vi "ReadSensorValues_v1.2.vi"(2 "VISA resource name":refnum<visa-resource-name>, 3 "Sensor type":T1) -> ()   [LabVIEW 2012]
uses:
  <vilib>/nican/nicantsk.llb/CAN Interface.ctl
  SensorTypes.ctl
  SensorStates.ctl
  <vilib>/nican/nicantsk.llb/CAN Task Reference.ctl
  <vilib>/nican/nicantsk.llb/CAN Mode.ctl
  globalVariables.vi
  <vilib>/Utility/file.llb/Write To Spreadsheet File (string).vi
  <vilib>/nican/nicantsk.llb/CAN Read Multi Chan Single Samp 1D Dbl.vi
  <instrlib>/Agilent 34970/Agilent 34970.lvlib
panel:
  in  "Cancel Measurement":bool
  out "new data":bool
  out "running":bool
  out "Sample number":i32
  in  "CAN Interface":T2 items=["CAN0"=0, "CAN1"=1, "CAN2"=2, "CAN3"=3, "CAN4"=4, "CAN5"=5, "CAN6"=6, "CAN7"=7, "CAN8"=8, "CAN9"=9, "CAN10"=10, "CAN11"=11, "CAN12"=12, "CAN13"=13, "CAN14"=14, "CAN15"=15, "CAN16"=16, "CAN17"=17, "CAN18"=18, "CAN19"=19, "CAN20"=20, "CAN21"=21, "CAN22"=22, "CAN23"=23, "CAN24"=24, "CAN25"=25, "CAN26"=26, "CAN27"=27, "CAN28"=28, "CAN29"=29, "CAN30"=30, "CAN31"=31, "CAN32"=32, "CAN33"=33, "CAN34"=34, "CAN35"=35, "CAN36"=36, "CAN37"=37, "CAN38"=38, "CAN39"=39, "CAN40"=40, "CAN41"=41, "CAN42"=42, "CAN43"=43, "CAN44"=44, "CAN45"=45, "CAN46"=46, "CAN47"=47, "CAN48"=48, "CAN49"=49, "CAN50"=50, "CAN51"=51, "CAN52"=52, "CAN53"=53, "CAN54"=54, "CAN55"=55, "CAN56"=56, "CAN57"=57, "CAN58"=58, "CAN59"=59, "CAN60"=60, "CAN61"=61, "CAN62"=62, "CAN63"=63, "MAX default"=64, "CAN256 (Virtual)"=256, "CAN257 (Virtual)"=257]
  out "Error Flag":bool
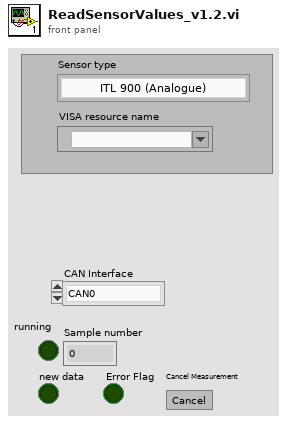
[diagram p1: front panel]
types:
  T1 = typedef "SensorTypes.ctl" = enum16{"ITL 900 (Analogue)", "CAB 300-C SP3 (CAN)", "xyz TODO (PWM)", "xyz TODO (LIN)", "xyz TODO (Analogue)"}
  T2 = typedef "CAN Interface.ctl" = u16
  T3 = typedef "SensorStates.ctl" = enum16{"init", "measure", "terminate"}
  T4 = cluster{"Include Alarm Data F:(No)":bool, "Include Channel # (F:No)":bool, "Include Time (F:No)":bool, "Include Units (F:No)":bool}
  T5 = cluster{"Aperture Value (.4)":dbl, "Aperture (1:Minimum)":u16, "NPLC (1)":u16, "Bandwidth (3 Hz)":u16, "Input Impedance (F:Fixed)":bool, "Integration Time (F:Aperture)":bool}
  T6 = enum16{"100 mV", "1 V", "10 V", "100 V", "300 V", "Minimum", "Maximum"}
  T7 = enum16{"Bus", "Immediate", "External", "Alarm 1", "Alarm 2", "Alarm 3", "Alarm 4", "Timer"}
  T8 = cluster{"Timeout Value (10000)":u32, "Baud Rate (57600)":enum16{"1200", "2400", "4800", "9600", "19200", "38400", "57600", "115200"}, "Flow Control (1:XON/XOFF)":enum16{"None", "XON / XOFF", "RTS / CTS", "DTR / DSR"}}
  T9 = typedef "CAN Task Reference.ctl" = u32
  T10 = enum16{"Remote Trigger", "Immediate Trigger", "Wait for Trigger", "Abort Scan"}
  T11 = typedef "CAN Mode.ctl" = u16
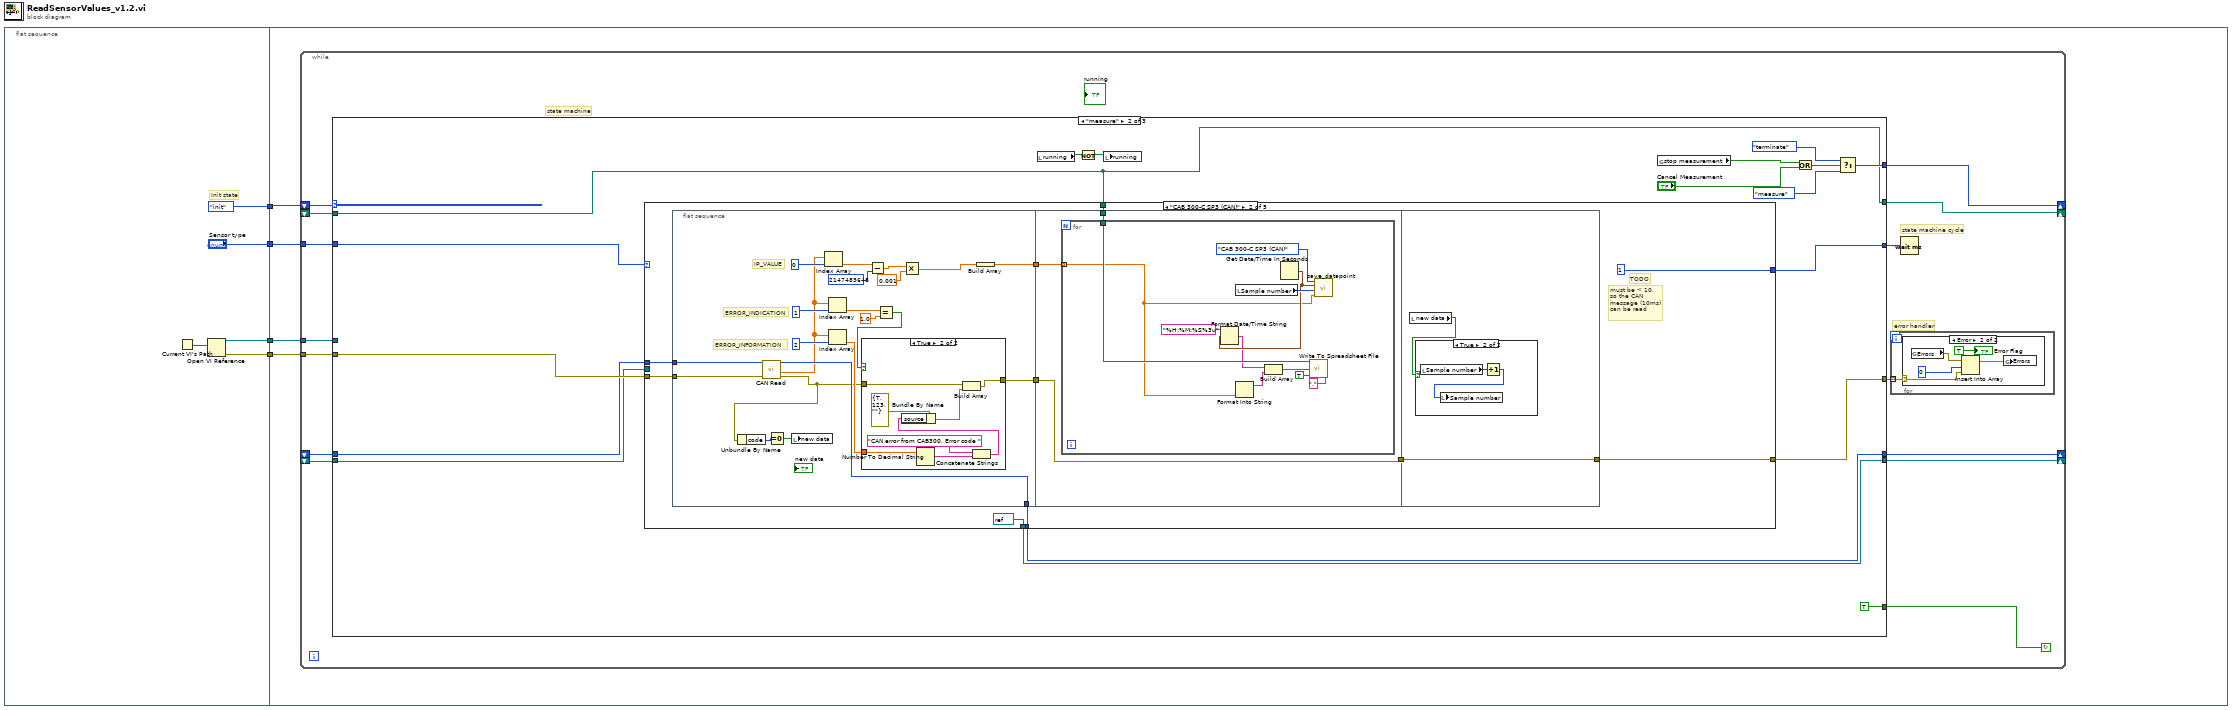
[diagram p0: block diagram]
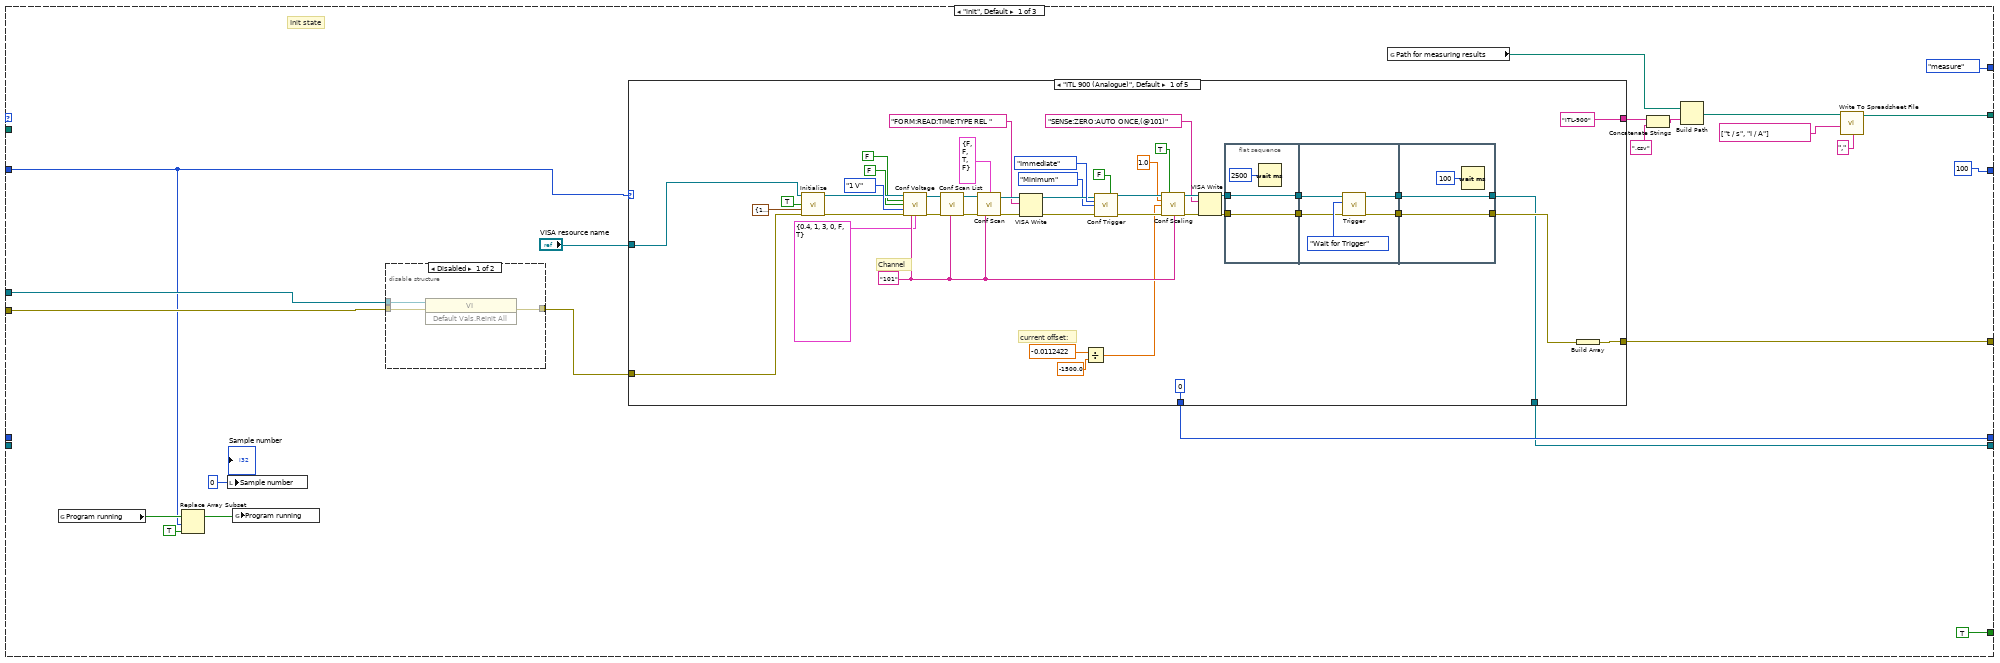
[diagram p3: hidden frame]
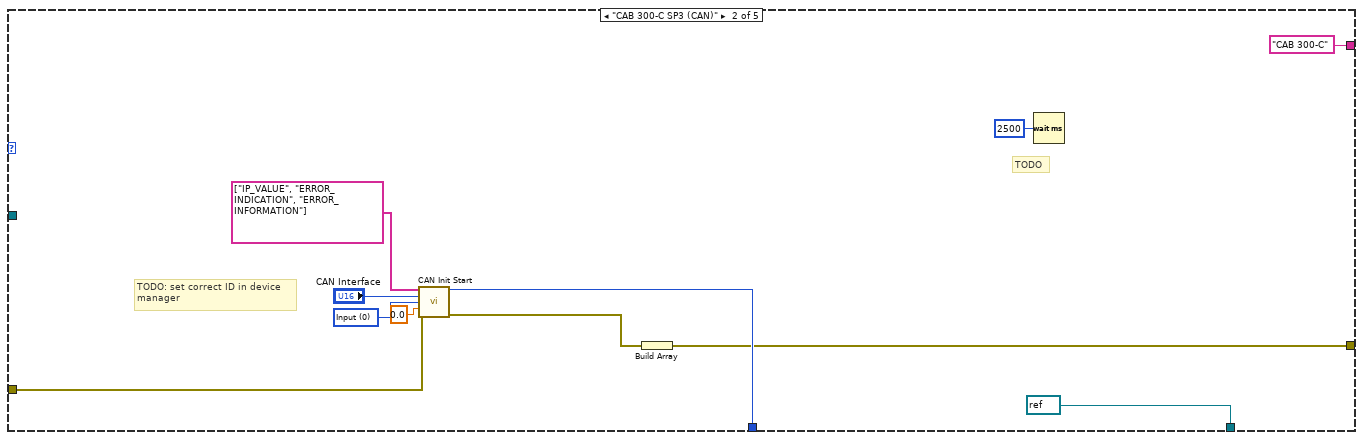
[diagram p5: hidden frame]
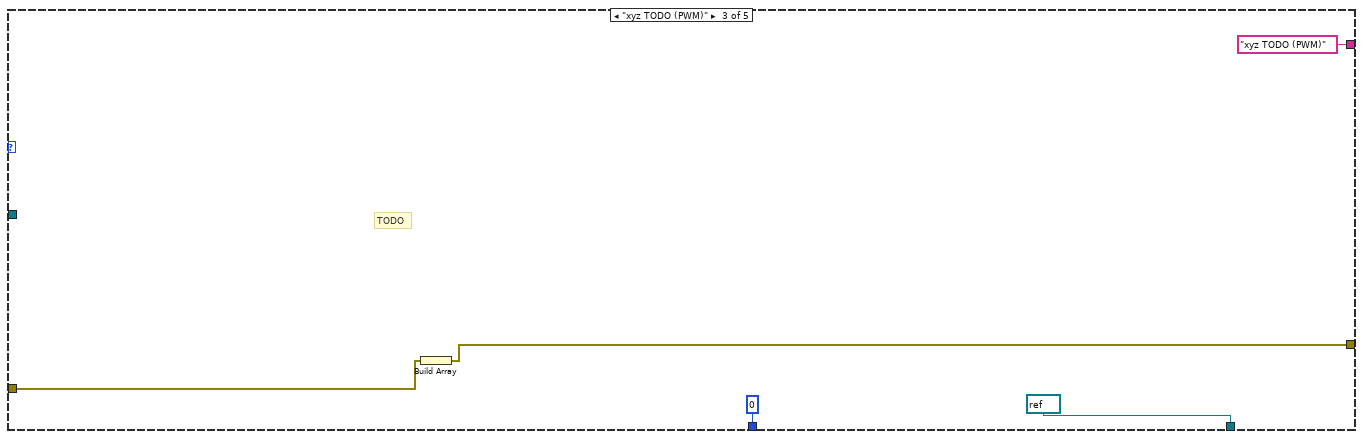
[diagram p6: hidden frame]
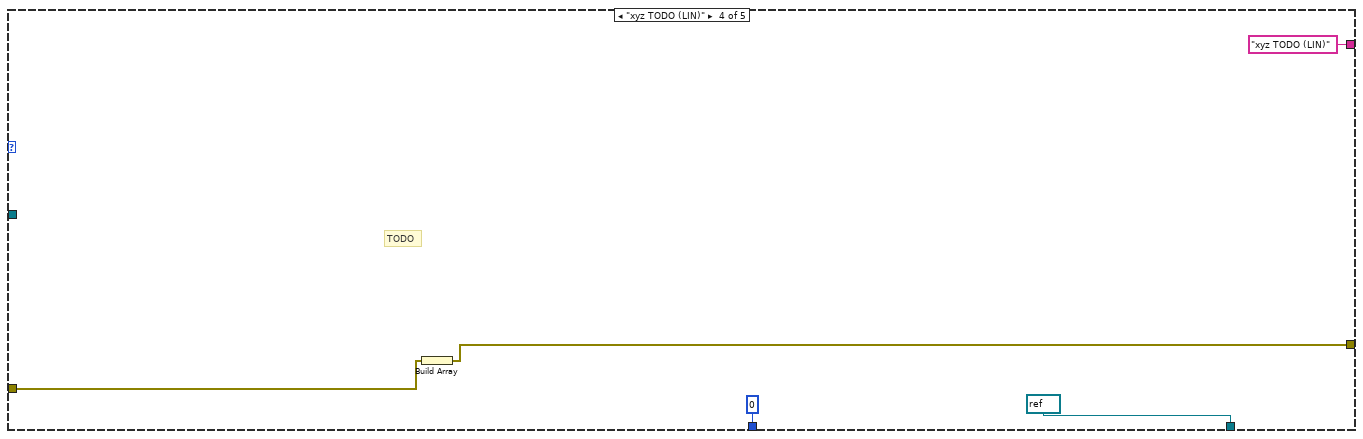
[diagram p7: hidden frame]
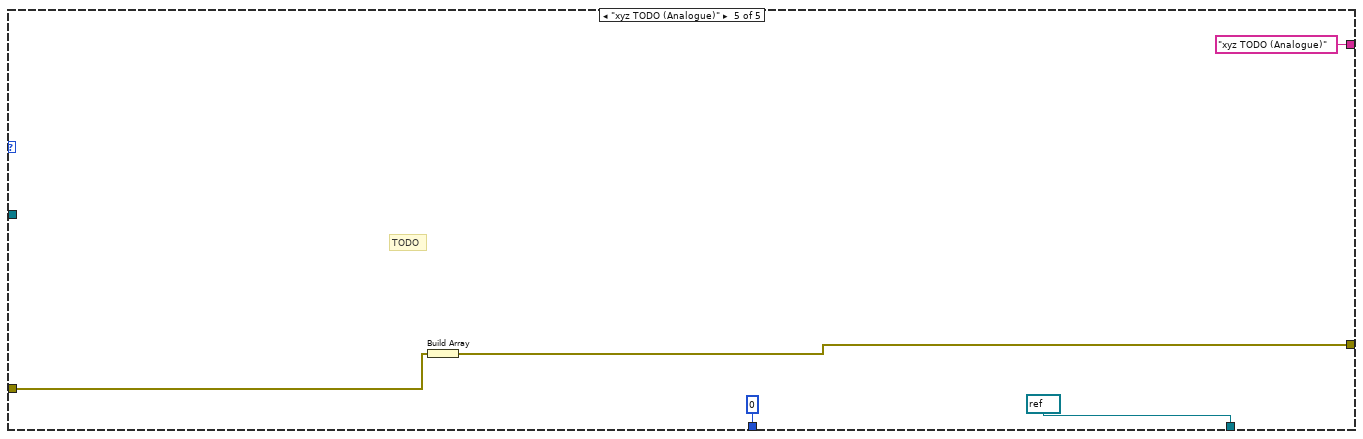
[diagram p8: hidden frame]
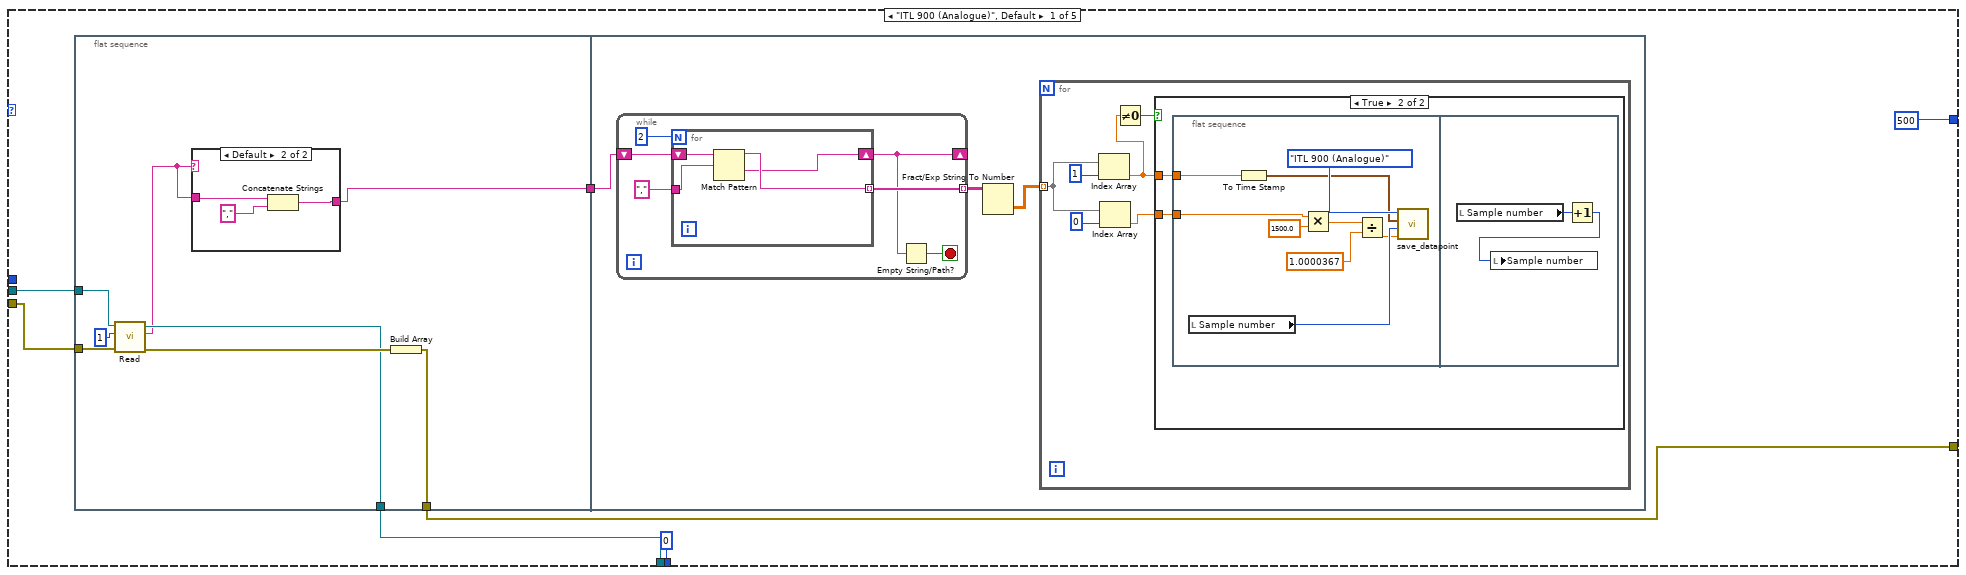
[diagram p9: hidden frame]
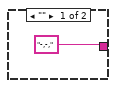
[diagram p10: hidden frame]
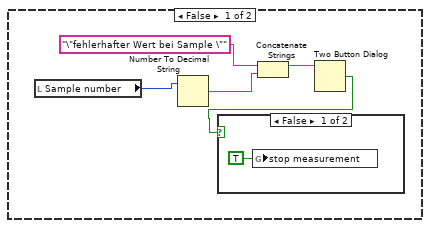
[diagram p11: hidden frame]
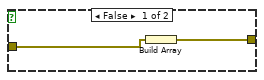
[diagram p13: hidden frame]
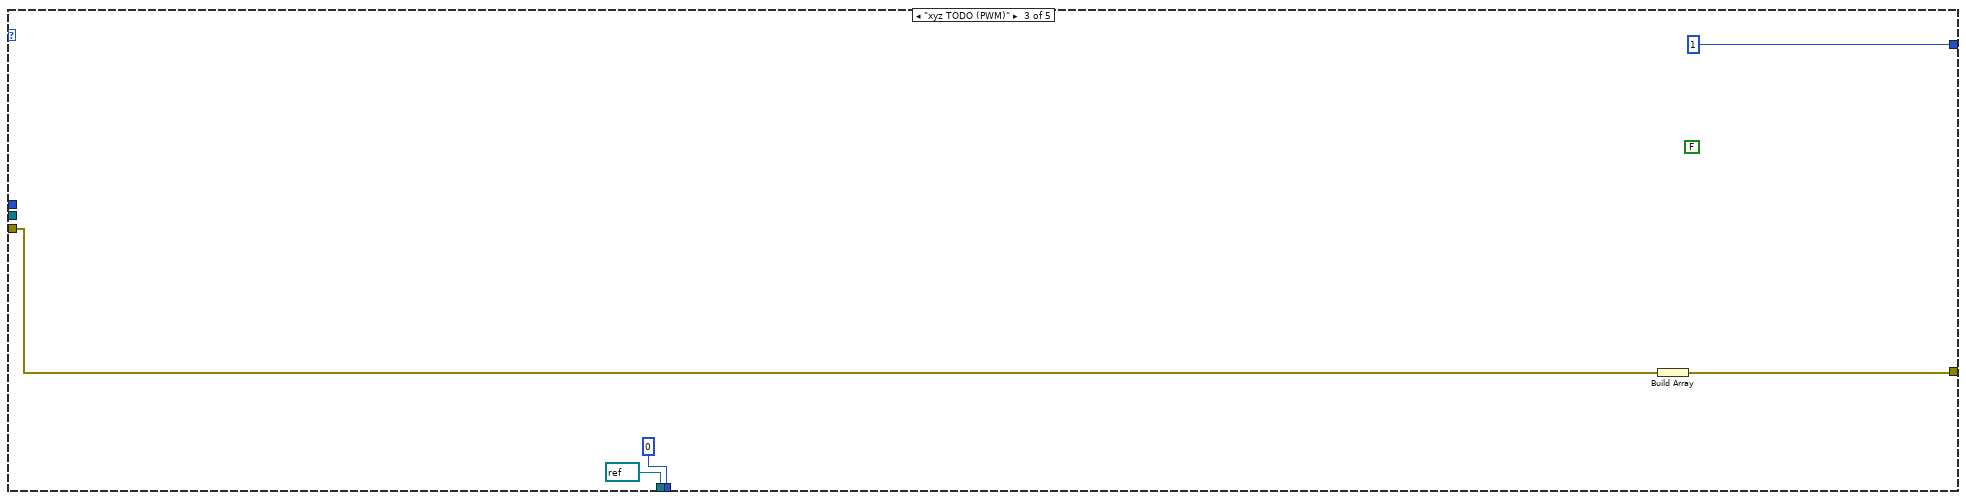
[diagram p15: hidden frame]
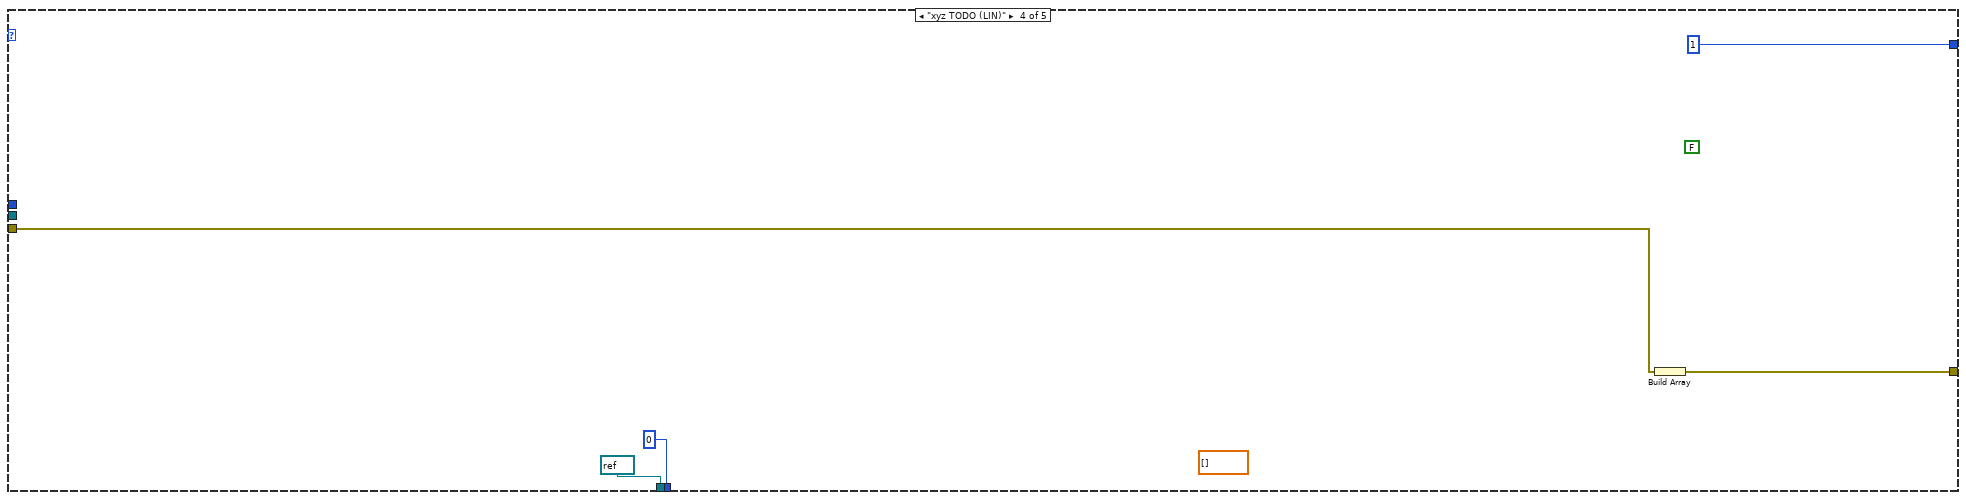
[diagram p16: hidden frame]
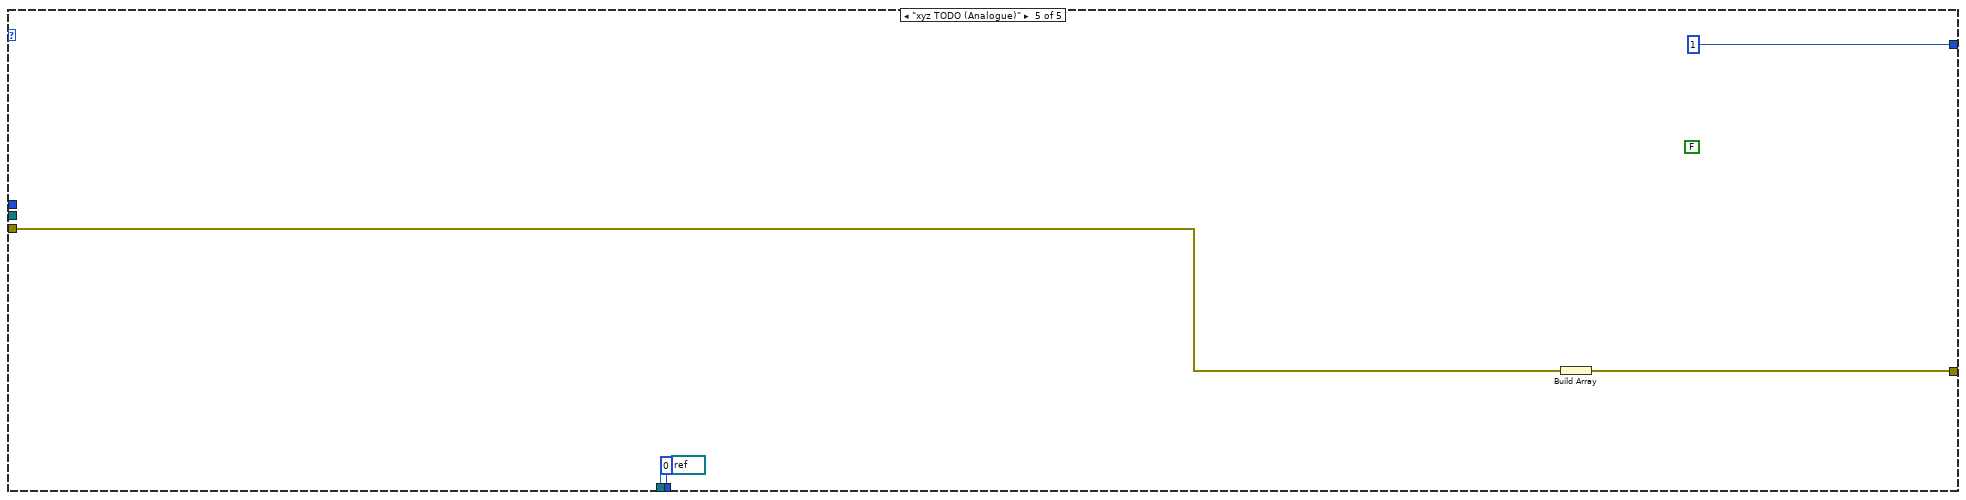
[diagram p17: hidden frame]
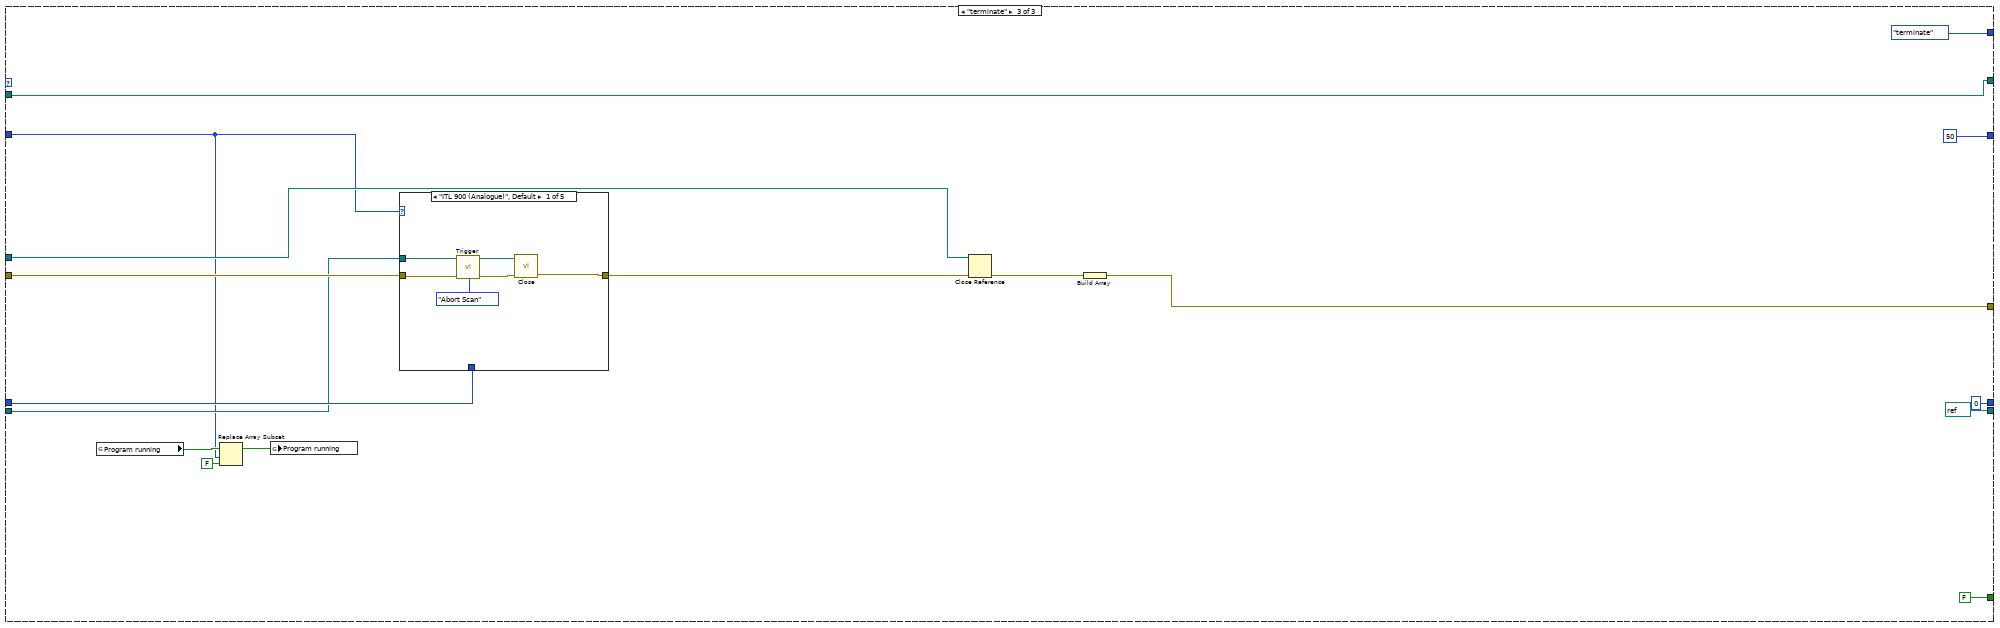
[diagram p18: hidden frame]
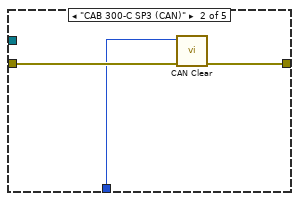
[diagram p19: hidden frame]
diagram:
  n1 = flat-sequence {
    tunnel: [SensorStates."init" ("States IEEE-488")] -> w4
    tunnel: [w9] -> w3
    tunnel: [w8] -> w2
    tunnel: ["Sensor type"] -> w1
    tunnel: w4 -> [w11]
    tunnel: w3 -> [w13]
    tunnel: w2 -> [w12]
    tunnel: w1 -> [w10]
    frame #0 {
      # "Init state"
      n2 = Current VI's Path() -> (path=w7:path)
      n3 = Open VI Reference(vi path=w7) -> (vi reference=w9:refnum<vi>, error out=w8:errorcluster)  [unwired: 2 in, 3 out]
    }
    frame #1 {
      n4 = while {
        tunnel: w13 -> [w26]
        tunnel: w12 -> [w25]
        shift-right: [w23] -> _
        shift-left: w11 -> [w24]
        shift-right: [w22] -> _
        shift-left: _ -> [w21]
        tunnel: w10 -> [w19]
        shift-right: [w18] -> _
        shift-left: _ -> [w17]
        shift-right: [w15] -> _
        shift-left: _ -> [w14]
        stop <- w16 continue-if-true
        # "state machine"
        # "error handler"
        # "state machine cycle"
        n5 = case shown="\"measure\"" w24 {
          tunnel: [u32 100 ("milliseconds to wait") w143 u32 50 ("milliseconds to wait")] -> w27
          tunnel: w26 -> [w54 _ w300]
          tunnel: w25 -> [w55 w156 w304]
          tunnel: [SensorStates."measure" ("States IEEE-488") w157 SensorStates."terminate" ("States IEEE-488")] -> w23
          tunnel: [w52 w150 T9 0 ("task reference out")] -> w22
          tunnel: w21 -> [_ w151 w303]
          tunnel: [w50 w152 w302] -> w20
          tunnel: w19 -> [w42 w144 w292]
          tunnel: [TRUE TRUE FALSE] -> w16
          tunnel: [w46 w145 refnum<visa-resource-name> refnum ("VISA Resource Name Out")] -> w18
          tunnel: w17 -> [_ w146 w297]
          tunnel: [w37 w142 w291] -> w15
          tunnel: w14 -> [_ w142 w291]
          frame "init", Default {
            # "Init state"
            n6 = global read "globalVariables.vi" "Program running"() -> (w45:bool[])
            n7 = Replace Array Subset(array=w45, new element=TRUE ("new element/subarray"), index=w42) -> (w44:bool[])
            n8 = local write "Sample number"(0 ("Sample number")) -> ()
            n9 = global write "globalVariables.vi" "Program running"(w44) -> ()
            n10 = disable-structure shown="Disabled" {
              disable-tunnel: w55 -> [w59 _]
              disable-tunnel: w54 -> [w58 _]
              disable-tunnel: [w57 _] -> w51
              frame Disabled {
                n11 = invoke class="VI" method="Default Vals.Reinit All"(reference=w58, error in=w59) -> (error out=w57:errorcluster)  [unwired: 1 in, 2 out]
              }
              frame Enabled {
              }
            }
            n12 = case shown="\"ITL 900 (Analogue)\", Default" w42 {
              tunnel: [T9 0 ("task reference out") w122 T9 0 ("task reference out") T9 0 ("task reference out") T9 0 ("task reference out")] -> w52
              tunnel: w51 -> [w71 w121 w130 w135 w141]
              tunnel: [w104 w119 w131 w136 w140] -> w50
              tunnel: "VISA resource name" -> [w64 _ _ _ _]
              tunnel: [w69 refnum<visa-resource-name> refnum ("VISA Resource Name Out") refnum<visa-resource-name> refnum ("VISA Resource Name Out") refnum<visa-resource-name> refnum ("VISA Resource Name Out") refnum<visa-resource-name> refnum ("VISA Resource Name Out")] -> w46
              tunnel: ["ITL-900" ("name or relative path") "CAB 300-C" ("name or relative path") "xyz TODO (PWM)" ("name or relative path") "xyz TODO (LIN)" ("name or relative path") "xyz TODO (Analogue)" ("name or relative path")] -> w36
              frame "ITL 900 (Analogue)", Default {
                w77 = "101" ("Channel List (Volt.)")
                # "current offset:"
                # "Channel"
                n13 = call <instrlib>:"Initialize.vi"("VISA Resource Name"=w64, "Reset (T: Reset)"=TRUE, "Serial Port Configuration"=T8 {"Timeout Value (10000)"=10000, "Baud Rate (57600)"=enum."57600", "Flow Control (1:XON/XOFF)"=enum."XON / XOFF"}, "error in (no error)"=w71) -> ("VISA Resource Name Out"=w98:refnum<visa-resource-name>, "error out"=w95:errorcluster)  [unwired: 10 in]
                n14 = call <instrlib>:"Conf Voltage.vi"("VISA Resource Name"=w98, "AC/DC (F:DC)"=FALSE, "Autorange? (F:Off)"=FALSE, "Range (6:Max)"=T6."1 V" ("Range (Volt.)"), "error in (no error)"=w95, "Channel List (empty)"=w77, "Advanced Config"=T5 {"Aperture Value (.4)"=0.4, "Aperture (1:Minimum)"=1, "NPLC (1)"=3, "Bandwidth (3 Hz)"=0, "Input Impedance (F:Fixed)"=FALSE, "Integration Time (F:Aperture)"=TRUE}) -> ("VISA Resource Name Out"=w97:refnum<visa-resource-name>, "error out"=w92:errorcluster)  [unwired: 6 in, 1 out]
                n15 = call <instrlib>:"Conf Scan List.vi"("Scan List (empty)"=w77, "error in (no error)"=w92, "VISA Resource Name"=w97) -> ("error out"=w91:errorcluster, "VISA Resource Name Out"=w93:refnum<visa-resource-name>)  [unwired: 6 in, 1 out]
                n16 = call <instrlib>:"Conf Scan.vi"("VISA Resource Name"=w93, "error in (no error)"=w91, "Channel List (empty)"=w77, "Scan Fields"=T4 {"Include Alarm Data F:(No)"=FALSE, "Include Channel # (F:No)"=FALSE, "Include Time (F:No)"=TRUE, "Include Units (F:No)"=FALSE}) -> ("VISA Resource Name Out"=w88:refnum<visa-resource-name>, "error out"=w87:errorcluster)  [unwired: 9 in, 1 out]
                n17 = VISA Write(VISA resource name=w88, write buffer="FORM:READ:TIME:TYPE REL ", error in (no error)=w87) -> (VISA resource name out=w85:refnum<visa-resource-name>, error out=w86:errorcluster)  [unwired: 1 out]
                n18 = Divide(x=-0.0112422, y=-1500.0) -> (x/y=w61:dbl)
                n19 = call <instrlib>:"Conf Trigger.vi"("VISA Resource Name"=w85, "Wait for Trigger? (F:No)"=FALSE, "Source (1:Immediate)"=T7."Immediate", "Time-Scan Interval (1:Min)"=enum16{"Manual", "Minimum", "Maximum"}."Minimum", "error in (no error)"=w86) -> ("VISA Resource Name Out"=w80:refnum<visa-resource-name>, "error out"=w79:errorcluster)  [unwired: 8 in, 1 out]
                n20 = call <instrlib>:"Conf Scaling.vi"("VISA Resource Name"=w80, "Enable Scaling? (T:Enable)"=TRUE, "Gain (1)"=1.0, "Offset (0)"=w61, "error in (no error)"=w79, "Channel List (empty)"=w77) -> ("VISA Resource Name Out"=w76:refnum<visa-resource-name>, "error out"=w75:errorcluster)  [unwired: 7 in, 1 out]
                n21 = VISA Write(VISA resource name=w76, write buffer="SENSe:ZERO:AUTO ONCE,(@101)", error in (no error)=w75) -> (VISA resource name out=w74:refnum<visa-resource-name>, error out=w73:errorcluster)  [unwired: 1 out]
                n22 = flat-sequence {
                  tunnel: [w106] -> w102
                  tunnel: w74 -> [w106]
                  tunnel: [w105] -> w101
                  tunnel: w73 -> [w105]
                  tunnel: w102 -> [w109]
                  tunnel: w101 -> [w108]
                  tunnel: [w112] -> w67
                  tunnel: [w111] -> w66
                  tunnel: [w114] -> w70
                  tunnel: [w115] -> w69
                  tunnel: w67 -> [w115]
                  tunnel: w66 -> [w114]
                  frame #0 {
                    n23 = Wait (ms)(milliseconds to wait=u32 2500) -> ()  [unwired: 1 out]
                  }
                  frame #1 {
                    n24 = call <instrlib>:"Trigger.vi"("error in (no error)"=w108, "Command (0:Rem Trig)"=T10."Wait for Trigger", "VISA Resource Name"=w109) -> ("error out"=w111:errorcluster, "VISA Resource Name Out"=w112:refnum<visa-resource-name>)  [unwired: 7 in]
                  }
                  frame #2 {
                    n25 = Wait (ms)(milliseconds to wait=u32 100) -> ()  [unwired: 1 out]
                  }
                }
                n26 = Build Array(w70) -> (w104:errorcluster[])
              }
              frame "CAB 300-C SP3 (CAN)" {
                w123 = T11 0 items=["Input", "Output", "Timestamped Input", "Output Recent"] ("mode")
                # "TODO"
                # "TODO: set correct ID in device\nmanager"
                n27 = call <vilib>:"CAN Init Start.vi"("channel list"=string[] ["IP_VALUE", "ERROR_INDICATION", "ERROR_INFORMATION"] ("Channel List"), "interface"="CAN Interface", "mode"=w123, "sample rate"=0.0, "error in (no error)"=w121) -> ("task reference out"=w122:T9, "error out"=w120:errorcluster)  [unwired: 9 in]
                n28 = Build Array(w120) -> (w119:errorcluster[])
                n29 = Wait (ms)(milliseconds to wait=u32 2500) -> ()  [unwired: 1 out]
              }
              frame "xyz TODO (PWM)" {
                # "TODO"
                n30 = Build Array(w130) -> (w131:errorcluster[])
              }
              frame "xyz TODO (LIN)" {
                # "TODO"
                n31 = Build Array(w135) -> (w136:errorcluster[])
              }
              frame "xyz TODO (Analogue)" {
                # "TODO"
                n32 = Build Array(w141) -> (w140:errorcluster[])
              }
            }
            n33 = global read "globalVariables.vi" "Path for measuring results"() -> (w38:path)
            n34 = Concatenate Strings(w36, ".csv" ("string")) -> (w34:string)
            n35 = Build Path(base path=w38, name or relative path=w34) -> (appended path=w39:path)
            n36 = call-poly <vilib>:"Write To Spreadsheet File.vi"("delimiter (\\t)"="," ("delimiter (\\t)"), "1D data"=string[] ["t / s", "I / A"], "file path (dialog if empty)"=w39) -> ("new file path (Not A Path if cancelled)"=w37:path)  [unwired: 5 in]
          }
          frame "measure" {
            n37 = case shown="\"CAB 300-C SP3 (CAN)\"" w144 {
              tunnel: w156 -> [w165 w223 w279 w283 w288]
              tunnel: [w162 w222 w280 w284 w289] -> w152
              tunnel: w151 -> [_ w221 _ _ _]
              tunnel: [T9 0 ("task reference out") w220 T9 0 ("task reference out") T9 0 ("task reference out") T9 0 ("task reference out")] -> w150
              tunnel: w146 -> [w166 _ _ _ _]
              tunnel: [w163 refnum<visa-resource-name> refnum ("VISA Resource Name Out") refnum<visa-resource-name> refnum ("VISA Resource Name Out") refnum<visa-resource-name> refnum ("VISA Resource Name Out") refnum<visa-resource-name> refnum ("VISA Resource Name Out")] -> w145
              tunnel: [u32 500 ("milliseconds to wait") u32 1 ("milliseconds to wait") u32 1 ("milliseconds to wait") u32 1 ("milliseconds to wait") u32 1 ("milliseconds to wait")] -> w143
              tunnel: w142 -> [_ w217 _ _ _]
              frame "ITL 900 (Analogue)", Default {
                n38 = flat-sequence {
                  tunnel: w166 -> [w172]
                  tunnel: w165 -> [w171]
                  tunnel: [w170] -> w164
                  tunnel: [w169] -> w163
                  tunnel: [w168] -> w162
                  tunnel: w164 -> [w181]
                  frame #0 {
                    n39 = call <instrlib>:"Read.vi"("error in (no error)"=w171, "# Channels (1)"=1, "VISA Resource Name"=w172) -> ("error out"=w173:errorcluster, "Readings"=w167:string, "VISA Resource Name Out"=w169:refnum<visa-resource-name>)  [unwired: 5 in, 1 out]
                    n40 = case shown="Default" w167 {
                      tunnel: ["-,-," ("string") w178] -> w170
                      tunnel: w167 -> [_ w177]
                      frame "" {
                      }
                      frame Default {
                        n41 = Concatenate Strings(w177, "," ("string")) -> (w178:string)
                      }
                    }
                    n42 = Build Array(w173) -> (w168:errorcluster[])
                  }
                  frame #1 {
                    n43 = while {
                      tunnel: [w186] -> w180 mode=indexing
                      shift-left: w181 -> [w187]
                      shift-right: [w183] -> _
                      stop <- w185 stop-if-true
                      n44 = for {
                        N: 2 -> [_]
                        tunnel: [w189] -> w186 mode=indexing
                        tunnel: "," ("regular expression") -> [w190]
                        shift-right: [w188] -> w183
                        shift-left: w187 -> [w191]
                        n45 = Match Pattern(string=w191, regular expression=w190) -> (before substring=w189:string, after substring=w188:string)  [unwired: 1 in, 2 out]
                      }
                      n46 = Empty String/Path?(string/path=w183) -> (empty?=w185:bool)
                    }
                    n47 = Fract/Exp String To Number(string=w180) -> (number=w179:dbl[][])  [unwired: 3 in, 1 out]
                    n48 = for {
                      tunnel: w179 -> [w195] mode=indexing
                      n49 = Index Array(array=w195, index=1 ("disabled index (col)")) -> (element=w192:dbl)
                      n50 = Index Array(array=w195, index=0 ("disabled index (col)")) -> (element=w194:dbl)
                      n51 = Not Equal To 0?(x=w192) -> (x != 0?=w193:bool)
                      n52 = case shown="True" w193 {
                        tunnel: w192 -> [_ w205]
                        tunnel: w194 -> [_ w204]
                        frame False {
                          n53 = local read "Sample number"() -> (w202:i32)
                          n54 = Number To Decimal String(number=w202) -> (decimal integer string=w199:string)  [unwired: 1 in]
                          n55 = Concatenate Strings("\"fehlerhafter Wert bei Sample \"" ("message"), w199) -> (w201:string)
                          n56 = Two Button Dialog(message=w201) -> (T button?=w198:bool)  [unwired: 2 in]
                          n57 = case shown="False" w198 {
                            frame False {
                              n58 = global write "globalVariables.vi" "stop measurement"(TRUE ("stop measurement")) -> ()
                            }
                            frame True {
                            }
                          }
                        }
                        frame True {
                          n59 = flat-sequence {
                            tunnel: w205 -> [w206]
                            tunnel: w204 -> [w207]
                            frame #0 {
                              n60 = local read "Sample number"() -> (w213:i32)
                              n61 = To Time Stamp(1:w206) -> (0:w208:timestamp)
                              n62 = Multiply(x=w207, y=1500.0) -> (x*y=w210:dbl)
                              n63 = Divide(x=w210, y=1.0000367) -> (x/y=w209:dbl)
                              n64 = call "save_datapoint.vi"("current value"=w209, "Sample number"=w213, "current time of measurement"=w208, "Sensor type"=SensorTypes."ITL 900 (Analogue)") -> ()
                            }
                            frame #1 {
                              n65 = local read "Sample number"() -> (w216:i32)
                              n66 = Increment(x=w216) -> (x+1=w215:i32)
                              n67 = local write "Sample number"(w215) -> ()
                            }
                          }
                        }
                      }
                    }
                  }
                }
              }
              frame "CAB 300-C SP3 (CAN)" {
                # "TODO"
                # "must be < 10,\nso the CAN \nmessage (10ms) \ncan be read"
                n68 = flat-sequence {
                  tunnel: [w246] -> w226
                  tunnel: [w245] -> w225
                  tunnel: w223 -> [w247]
                  tunnel: w221 -> [w244]
                  tunnel: [w243] -> w220
                  tunnel: w226 -> [w260]
                  tunnel: w225 -> [w259]
                  tunnel: [w260] -> w224
                  tunnel: w217 -> [w258]
                  tunnel: w224 -> [w273]
                  tunnel: [w273] -> w222
                  frame #0 {
                    # "ERROR_INFORMATION"
                    # "ERROR_INDICATION"
                    # "IP_VALUE"
                    n69 = call-poly <vilib>:"CAN Read.vi"("error in (no error)"=w247, "task reference in"=w244) -> ("error out"=w234:errorcluster, "multi-chan single-samp 1D dbl"=w237:dbl[], "task reference out"=w243:T9)  [unwired: 6 in, 1 out]
                    n70 = Unbundle By Name(w234) -> ("code"=w233:i32)
                    n71 = Equal To 0?(x=w233) -> (x = 0?=w232:bool)
                    n72 = local write "new data"(w232) -> ()
                    n73 = Index Array(array=w237, index=0) -> (element=w231:dbl)
                    n74 = Index Array(array=w237, index=1) -> (element=w239:dbl)
                    n75 = Index Array(array=w237, index=2) -> (element=w236:dbl)
                    n76 = Subtract(x=w231, y=u32 2147483648) -> (x-y=w229:dbl)
                    n77 = Equal?(x=w239, y=1.0) -> (x = y?=w235:bool)
                    n78 = case shown="True" w235 {
                      tunnel: w234 -> [w249 w257]
                      tunnel: [w248 w256] -> w246
                      tunnel: w236 -> [_ w251]
                      frame False {
                        n79 = Build Array(w249) -> (w248:errorcluster[])
                      }
                      frame True {
                        n80 = Number To Decimal String(number=w251) -> (decimal integer string=w252:string)  [unwired: 1 in]
                        n81 = Concatenate Strings("CAN error from CAB300. Error code ", w252) -> (w250:string)
                        n82 = Bundle By Name(cluster=errorcluster {"status"=TRUE, "code"=123, "source"=""} ("error out"), "source"=w250) -> (w254:errorcluster)
                        n83 = Build Array(w257, w254) -> (w256:errorcluster[])
                      }
                    }
                    n84 = Multiply(x=w229, y=0.001) -> (x*y=w227:dbl)
                    n85 = Build Array(w227) -> (w245:dbl[])
                  }
                  frame #1 {
                    n86 = for {
                      tunnel: w259 -> [w264] mode=indexing
                      tunnel: w258 -> [w269]
                      n87 = local read "Sample number"() -> (w270:i32)
                      n88 = Format Into String(w264) -> (resulting string=w263:string)  [unwired: 3 in, 1 out]
                      n89 = Get Date/Time In Seconds() -> (seconds since 1Jan1904=w267:timestamp)
                      n90 = Format Date/Time String(time format string (%c)="%H:%M:%S%3u", seconds (now)=w267) -> (date/time string=w266:string)  [unwired: 1 in]
                      n91 = Build Array(w266, w263) -> (w265:string[])
                      n92 = call-poly <vilib>:"Write To Spreadsheet File.vi"("delimiter (\\t)"="," ("delimiter (\\t)"), "append to file? (new file:F)"=TRUE, "1D data"=w265, "file path (dialog if empty)"=w269) -> ()  [unwired: 4 in, 1 out]
                      n93 = call "save_datapoint.vi"("current value"=w264, "Sample number"=w270, "current time of measurement"=w267, "Sensor type"=SensorTypes."CAB 300-C SP3 (CAN)") -> ()
                    }
                  }
                  frame #2 {
                    n94 = local read "new data"() -> (w272:bool)
                    n95 = case shown="True" w272 {
                      frame False {
                      }
                      frame True {
                        n96 = local read "Sample number"() -> (w275:i32)
                        n97 = Increment(x=w275) -> (x+1=w274:i32)
                        n98 = local write "Sample number"(w274) -> ()
                      }
                    }
                  }
                }
              }
              frame "xyz TODO (PWM)" {
                (unwired) FALSE ("new data")
                n99 = Build Array(w279) -> (w280:errorcluster[])
              }
              frame "xyz TODO (LIN)" {
                (unwired) dbl[] []
                (unwired) FALSE ("new data")
                n100 = Build Array(w283) -> (w284:errorcluster[])
              }
              frame "xyz TODO (Analogue)" {
                (unwired) FALSE ("new data")
                n101 = Build Array(w288) -> (w289:errorcluster[])
              }
            }
            n102 = local read "running"() -> (w154:bool)
            n103 = Not(x=w154) -> (.not. x?=w155:bool)
            n104 = local write "running"(w155) -> ()
            n105 = global read "globalVariables.vi" "stop measurement"() -> (w149:bool)
            n106 = Or(x=w149, y="Cancel Measurement") -> (x .or. y?=w147:bool)
            n107 = Select(t=SensorStates."terminate" ("States IEEE-488"), s=w147, f=SensorStates."measure" ("States IEEE-488")) -> (s? t:f=w157:T3)
          }
          frame "terminate" {
            n108 = global read "globalVariables.vi" "Program running"() -> (w295:bool[])
            n109 = Replace Array Subset(array=w295, new element=FALSE ("new element/subarray"), index=w292) -> (w294:bool[])
            n110 = global write "globalVariables.vi" "Program running"(w294) -> ()
            n111 = case shown="\"ITL 900 (Analogue)\", Default" w292 {
              tunnel: w304 -> [w310 w316 w317 w318 w319]
              tunnel: [w309 w315 w317 w318 w319] -> w299
              tunnel: w303 -> [_ w314 _ _ _]
              tunnel: w297 -> [w308 _ _ _ _]
              frame "ITL 900 (Analogue)", Default {
                n112 = call <instrlib>:"Trigger.vi"("error in (no error)"=w310, "Command (0:Rem Trig)"=T10."Abort Scan", "VISA Resource Name"=w308) -> ("error out"=w312:errorcluster, "VISA Resource Name Out"=w311:refnum<visa-resource-name>)  [unwired: 7 in]
                n113 = call <instrlib>:"Close.vi"("VISA Resource Name"=w311, "error in (no error)"=w312) -> ("error out"=w309:errorcluster)  [unwired: 13 in]
              }
              frame "CAB 300-C SP3 (CAN)" {
                n114 = call <vilib>:"CAN Clear.vi"("error in (no error)"=w316, "task reference in"=w314) -> ("error out"=w315:errorcluster)  [unwired: 9 in]
              }
              frame "xyz TODO (PWM)" {
              }
              frame "xyz TODO (LIN)" {
              }
              frame "xyz TODO (Analogue)" {
              }
            }
            n115 = Close Reference(reference=w300, error in (no error)=w299) -> (error out=w306:errorcluster)
            n116 = Build Array(w306) -> (w302:errorcluster[])
          }
        }
        n117 = for {
          tunnel: w20 -> [w28] mode=indexing
          n118 = case shown="Error" w28 {
            selector: w28 -> [_ w32]
            frame No Error {
            }
            frame Error {
              n119 = global read "globalVariables.vi" "Errors"() -> (w30:errorcluster[])
              n120 = Insert Into Array(array=w30, index=0, new element=w32) -> (w29:errorcluster[])
              n121 = global write "globalVariables.vi" "Errors"(w29) -> ()
              "Error Flag" <- TRUE ("Error Flag")
            }
          }
        }
        n122 = Wait (ms)(milliseconds to wait=w27) -> ()  [unwired: 1 out]
      }
    }
  }
